vi "test Data Retrieval.vi"(8 "error in (no error)":errorcluster, 11 "BM Data in":refnum<class "BM Data.lvclass">) -> (0 "error out":errorcluster, 3 "BM Data out":refnum<class "BM Data.lvclass">)   [LabVIEW 2016, in "BM Data.lvclass"]
uses:
  BM Data.lvclass
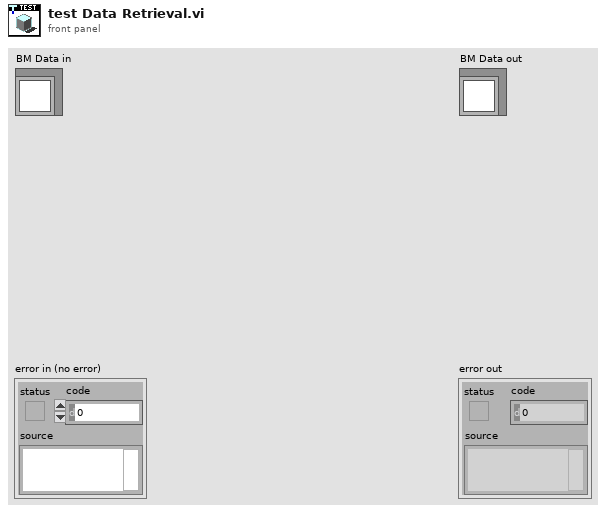
[diagram p1: front panel]
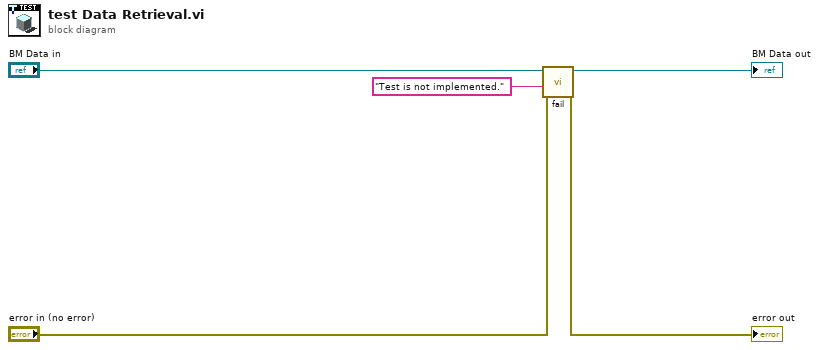
[diagram p0: block diagram]
diagram:
  n1 = call-dynamic "fail.vi"("error in (no error)"="error in (no error)", "message (\"\")"="Test is not implemented." ("message (\"\")"), "TestCase in"="BM Data in") -> ("error out"=→"error out":errorcluster, "TestCase out"=→"BM Data out":refnum<class "BM Data.lvclass">)  [unwired: 7 in]
